vi "Cmd Set Parameter Value (C).vi"(6 "error in (no error)":errorcluster, 7 "value":variant, 8 "parameter index":variant, 9 "command reference":T1) -> (0 "error out":errorcluster, 3 "command reference out":T1)   [LabVIEW 2017, in "NI_Database_API.lvlib"]
doc: "Sets the value of the parameter at <B>parameter index</B> in the command or command-recordset. The <B>parameter index</B> can be either the zero-indexed position of the parameter in the command or the name of the parameter. Wire data to the reference input to determine the polymorphic instance to use or manually select the instance."
uses:
  <vilib>/addons/database/NI_Database_API.lvlib
  <vilib>/addons/database/Command.llb/Cmd ObjectReference.ctl
  <vilib>/Utility/VariantDataType/VariantType.lvlib
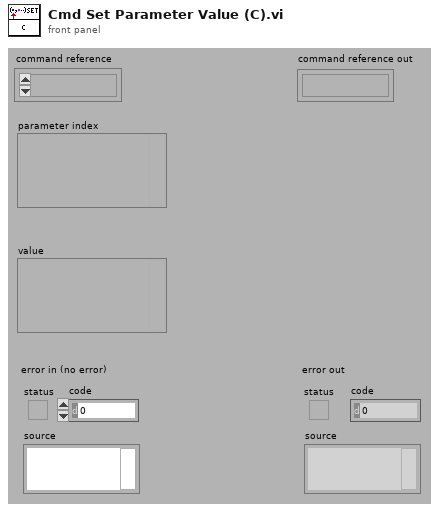
[diagram p1: front panel]
types:
  T1 = typedef "NI_Database_API.lvlib/Cmd ObjectReference.ctl" = refnum<k1>
  T2 = typedef "VariantType.lvlib/Type.ctl" = enum8{"Invalid Type", "Void", "I8", "I16", "I32", "I64", "U8", "U16", "U32", "U64", "Single Float", "Double Float", "Extended Float", "Single Complex", "Double Complex", "Extended Complex", "Enum U8", "Enum U16", "Enum U32", "Enum U64", "Single Float With Unit", "Double Float With Unit", "Extended Float With Unit", "Single Complex with Unit", "Double Complex with Unit", "Extended Complex with Unit", "Boolean", "String", "Path", "Picture", "Tag", "Array", "Cluster", "Variant", "LV Variant", "Waveform", "Timestamp", "Digital Waveform", "Digital Data", "ExpressData", "Refnum", "External Data", "VI", "Poly VI", "LabVIEW Class Instance", "Fixed Point"}
  T3 = typedef "NI_Database_API.lvlib/DB Tools DataTypes.ctl" = enum16{"String", "Long (I32)", "Single (SGL)", "Double (DBL)", "Date/Time", "Binary"}
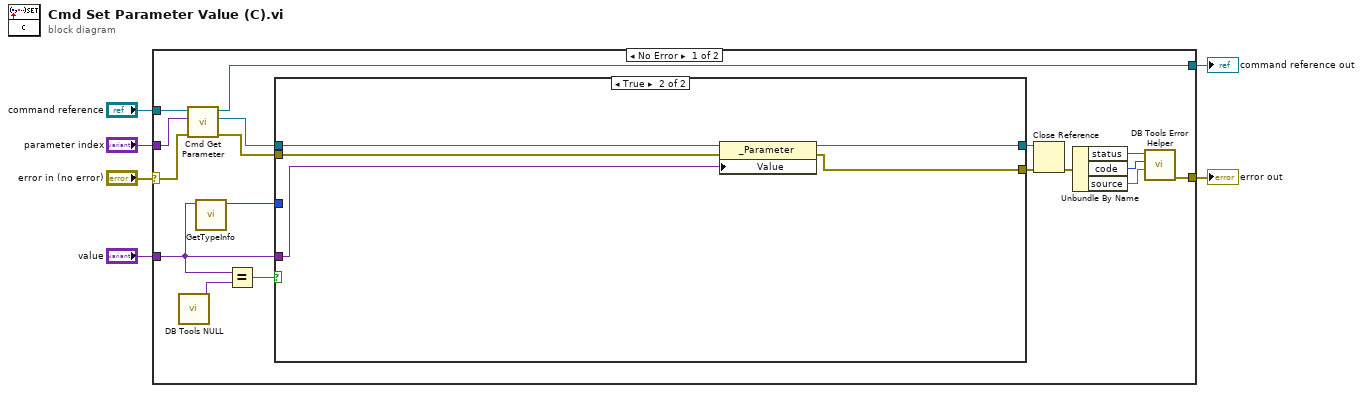
[diagram p0: block diagram]
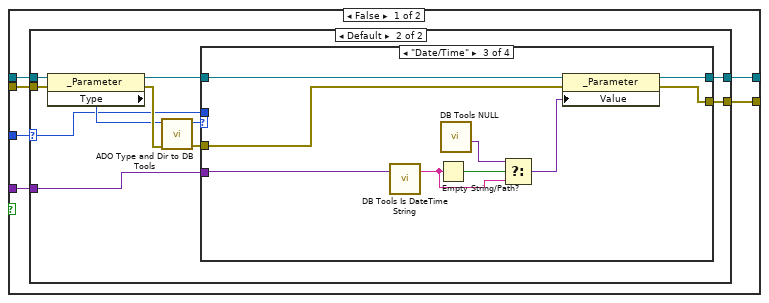
[diagram p2: hidden frame]
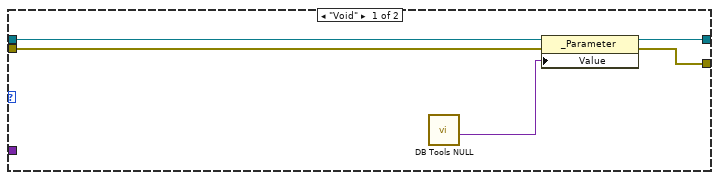
[diagram p3: hidden frame]
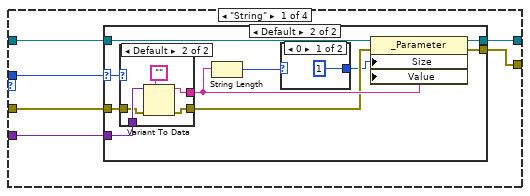
[diagram p4: hidden frame]
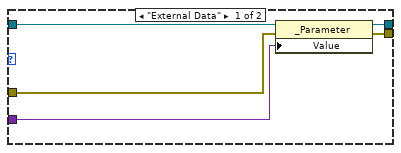
[diagram p5: hidden frame]
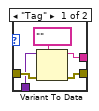
[diagram p7: hidden frame]
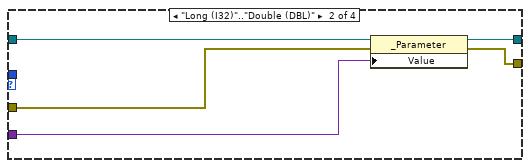
[diagram p8: hidden frame]
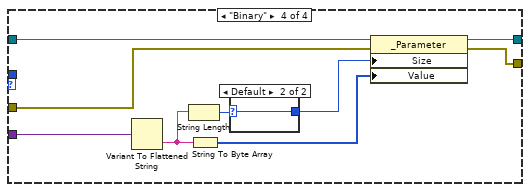
[diagram p9: hidden frame]
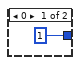
[diagram p10: hidden frame]
diagram:
  n1 = case shown="No Error" "error in (no error)" {
    selector: "error in (no error)" -> [w15 w110]
    tunnel: "value" -> [w10 _]
    tunnel: "command reference" -> [w23 w109]
    tunnel: "parameter index" -> [w22 _]
    tunnel: [w21 w109] -> w3
    tunnel: [w16 w110] -> w2
    frame No Error {
      n2 = call <vilib>:"DB Tools NULL.vi"() -> ("NULL"=w14:variant)  [unwired: 10 in, 1 out]
      n3 = call <vilib>:"Cmd Get Parameter.vi"("error in (no error)"=w15, "parameter index"=w22, "command reference"=w23) -> ("error out"=w7:errorcluster, "ADODB.Parameter"=w8:refnum<k7>, "command reference out"=w21:T1)  [unwired: 2 out]
      n4 = call <vilib>:"GetTypeInfo.vi"("Variant"=w10) -> ("Type Enum"=w9:T2)  [unwired: 1 in, 9 out]
      n5 = Equal?(x=w10, y=w14) -> (x = y?=w11:bool)
      n6 = case shown="True" w11 {
        tunnel: [w29 w106] -> w13
        tunnel: [w28 w105] -> w12
        tunnel: w10 -> [w27 w104]
        tunnel: w9 -> [w26 _]
        tunnel: w8 -> [w25 w108]
        tunnel: w7 -> [w24 w107]
        frame False {
          n7 = case shown="Default" w26 {
            selector: w26 -> [_ w35]
            tunnel: [w34 w45] -> w29
            tunnel: [w31 w44] -> w28
            tunnel: w25 -> [w33 w42]
            tunnel: w24 -> [w32 w41]
            tunnel: w27 -> [_ w36]
            frame "Void" {
              n8 = call <vilib>:"DB Tools NULL.vi"() -> ("NULL"=w30:variant)  [unwired: 10 in, 1 out]
              n9 = property class="_Parameter"(reference=w33, error in=w32, "Value"=w30) -> (reference out=w34:refnum<k7>, error out=w31:errorcluster)
            }
            frame Default {
              n10 = property class="_Parameter"(reference=w42, error in=w41) -> (reference out=w43:refnum<k7>, error out=w40:errorcluster, "Type"=w39:i32)
              n11 = call <vilib>:"ADO Type and Dir to DB Tools.vi"("error in (no error)"=w40, "ADO type"=w39) -> ("error out"=w37:errorcluster, "data type"=w38:T3)  [unwired: 1 in, 3 out]
              n12 = case shown="\"Date/Time\"" w38 {
                tunnel: w36 -> [w48 w80 w88 w100]
                tunnel: [w51 w83 w92 w99] -> w45
                tunnel: [w50 w82 w91 w98] -> w44
                tunnel: w43 -> [w49 w81 w84 w97]
                tunnel: w37 -> [w47 w79 w89 w95]
                tunnel: w35 -> [w46 _ _ _]
                frame "String" {
                  n13 = case shown="Default" w46 {
                    selector: w46 -> [_ w57]
                    tunnel: [w55 w66] -> w51
                    tunnel: [w52 w65] -> w50
                    tunnel: w49 -> [w56 w64]
                    tunnel: w48 -> [w54 w61]
                    tunnel: w47 -> [w53 w60]
                    frame "External Data" {
                      n14 = property class="_Parameter"(reference=w56, error in=w53, "Value"=w54) -> (reference out=w55:refnum<k7>, error out=w52:errorcluster)
                    }
                    frame Default {
                      n15 = case shown="Default" w57 {
                        tunnel: [w70 w77] -> w63
                        tunnel: [w72 w76] -> w62
                        tunnel: w60 -> [w73 w74]
                        tunnel: w61 -> [w71 w75]
                        frame "Tag" {
                          n16 = Variant To Data(error in=w73, type=tag "", Variant=w71) -> (data=w70:tag, error out=w72:errorcluster)
                        }
                        frame Default {
                          n17 = Variant To Data(error in=w74, type="", Variant=w75) -> (data=w77:string, error out=w76:errorcluster)
                        }
                      }
                      n18 = String Length(string=w63) -> (length=w59:i32)
                      n19 = case shown="0" w59 {
                        selector: w59 -> [_ w68]
                        tunnel: [1 w68] -> w58
                        frame 0 {
                        }
                        frame Default {
                        }
                      }
                      n20 = property class="_Parameter"(reference=w64, error in=w62, "Size"=w58, "Value"=w63) -> (reference out=w66:refnum<k7>, error out=w65:errorcluster)
                    }
                  }
                }
                frame "Long (I32)".."Double (DBL)" {
                  n21 = property class="_Parameter"(reference=w81, error in=w79, "Value"=w80) -> (reference out=w83:refnum<k7>, error out=w82:errorcluster)
                }
                frame "Date/Time" {
                  n22 = call <vilib>:"DB Tools Is DateTime String.vi"("string or date/time"=w88) -> ("data"=w85:string)  [unwired: 2 out]
                  n23 = Empty String/Path?(string/path=w85) -> (empty?=w87:bool)
                  n24 = call <vilib>:"DB Tools NULL.vi"() -> ("NULL"=w86:variant)  [unwired: 10 in, 1 out]
                  n25 = Select(t=w86, s=w87, f=w85) -> (s? t:f=w90:variant)
                  n26 = property class="_Parameter"(reference=w84, error in=w89, "Value"=w90) -> (reference out=w92:refnum<k7>, error out=w91:errorcluster)
                }
                frame "Binary" {
                  n27 = Variant To Flattened String(Variant=w100) -> (data string=w101:string)  [unwired: 1 out]
                  n28 = String Length(string=w101) -> (length=w94:i32)
                  n29 = String To Byte Array(string=w101) -> (unsigned byte array=w96:u8[])
                  n30 = case shown="Default" w94 {
                    selector: w94 -> [_ w103]
                    tunnel: [1 w103] -> w93
                    frame 0 {
                    }
                    frame Default {
                    }
                  }
                  n31 = property class="_Parameter"(reference=w97, error in=w95, "Size"=w93, "Value"=w96) -> (reference out=w99:refnum<k7>, error out=w98:errorcluster)
                }
              }
            }
          }
        }
        frame True {
          n32 = property class="_Parameter"(reference=w108, error in=w107, "Value"=w104) -> (reference out=w106:refnum<k7>, error out=w105:errorcluster)
        }
      }
      n33 = Close Reference(reference=w13, error in (no error)=w12) -> (error out=w17:errorcluster)
      n34 = Unbundle By Name(w17) -> ("status"=w19:bool, "code"=w18:i32, "source"=w20:string)
      n35 = call <vilib>:"DB Tools Error Helper.vi"("source"=w20, "code"=w18, "status"=w19) -> ("error out"=w16:errorcluster)  [unwired: 1 in, 7 out]
    }
    frame Error {
    }
  }
  "error out" <- w2
  "command reference out" <- w3
